vi "PKYK_Status.vi"(4 "QUpdate":bool=TRUE, 6 "PokaYoke?":bool, 8 "error in (no error)":errorcluster, 11 "Ref in":T5={"MS SQL Connection"=refnum, "UDL File"=path "", "Time"="", "DCODE"="", "WIP+1"=0, "MC No?"=0, "POKAYOKE?"=FALSE, "Expected Result"="", "Result [Status]"="", "Clock"=0.0, "RFID"="", "WIP Queue"=refnum, "TS Parameter"={"ProfitCenterCode"="", "LineCode"="", "WorkOrderNumber"="", "Model"="", "Model_with_Prefix"="", "VendorCode"="", "SetParameterDateCode"="", "PokaYoke"=0, "Target"=1, "Live_DateCode"="", "CustomerPartNumber"="", "Hand"="", "sBarcode"=FALSE, "FCA"=0, "Ent_Stamp"=timestamp(0 s since 1904-01-01), "STS_CD"=0.0}, "Data_Queue"=[], "RFID Serial No."=""} {"TS Parameter"."FCA" format="%01d"; "TS Parameter"."Target" min=1 max=100000; "TS Parameter"."PokaYoke" min=0 max=1}) -> (0 "error out":errorcluster, 2 "PKYK_Data Out":T1, 3 "Ref out":T5={"MS SQL Connection"=refnum, "UDL File"=path "", "Time"="", "DCODE"="", "WIP+1"=0, "MC No?"=0, "POKAYOKE?"=FALSE, "Expected Result"="", "Result [Status]"="", "Clock"=0.0, "RFID"="", "WIP Queue"=refnum, "TS Parameter"={"ProfitCenterCode"="", "LineCode"="", "WorkOrderNumber"="", "Model"="", "Model_with_Prefix"="", "VendorCode"="", "SetParameterDateCode"="", "PokaYoke"=0, "Target"=1, "Live_DateCode"="", "CustomerPartNumber"="", "Hand"="", "sBarcode"=FALSE, "FCA"=0, "Ent_Stamp"=timestamp(0 s since 1904-01-01), "STS_CD"=0.0}, "Data_Queue"=[], "RFID Serial No."=""} {"TS Parameter"."FCA" format="%01d"; "TS Parameter"."Target" min=1 max=100000; "TS Parameter"."PokaYoke" min=0 max=1}, 5 "Pky Status":T2)   [LabVIEW 2020]
uses:
  Controls/TD SQL.ctl
  <vilib>/addons/database/Connection.llb/Conn ObjectReference.ctl
  Controls/WIP_State.ctl
  Controls/TS_Parameter.ctl
  Controls/Poka_Status.ctl
  Controls/PKYK_qData.ctl
  Controls/PKYK_Barcode_Status.ctl
  Controls/PKYK_Status.ctl
  <vilib>/addons/database/NI_Database_API.lvlib
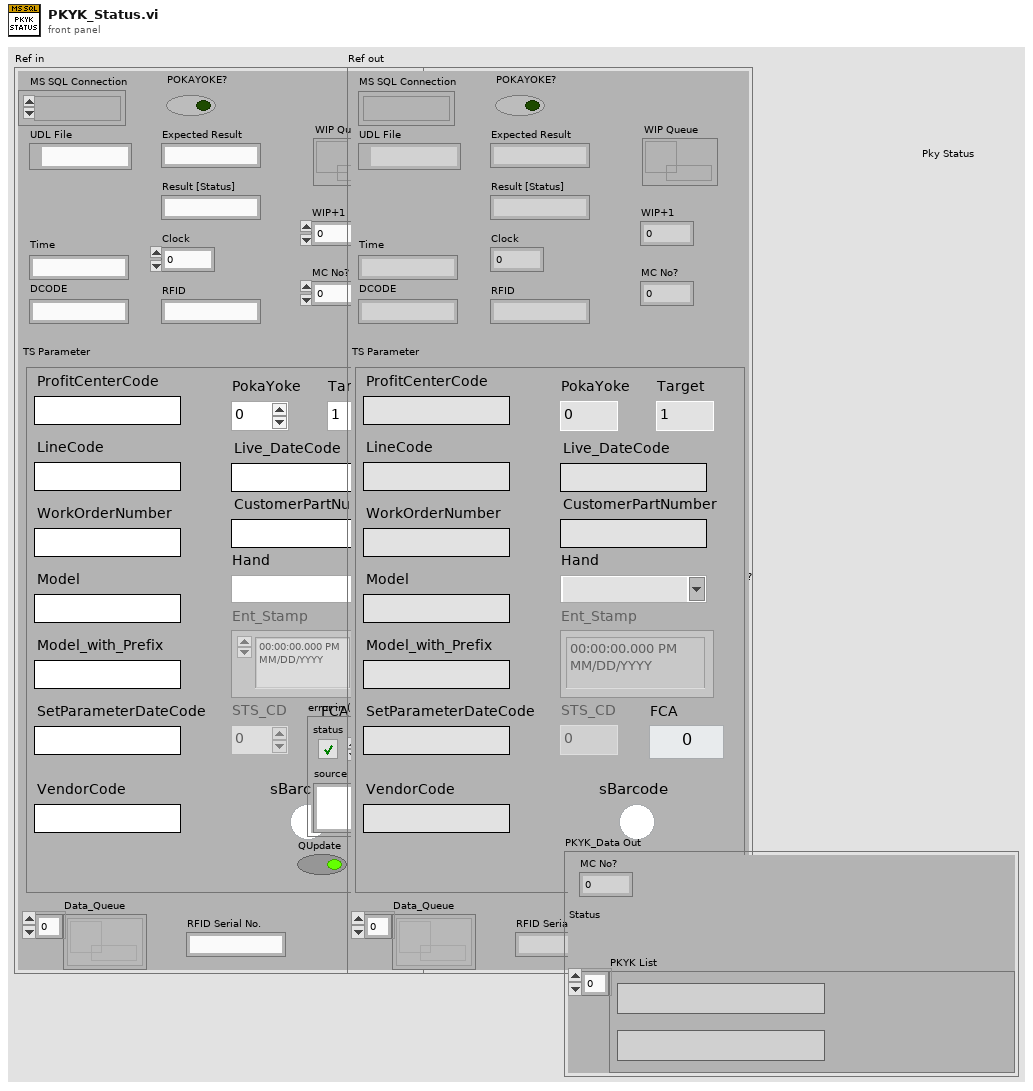
[diagram p1: front panel]
types:
  T1 = typedef "PKYK_qData.ctl" = cluster{"MC No?":i32, "Status":T2, "PKYK List":T3[]}
  T2 = typedef "Poka_Status.ctl" = u16
  T3 = typedef "PKYK_Barcode_Status.ctl" = cluster{"RFID Written Last":string, "Result":T4, "Exp. Result":T4}
  T4 = typedef "PKYK_Status.ctl" = u16
  T5 = typedef "TD SQL.ctl" = cluster{"MS SQL Connection":T6, "UDL File":path, "Time":string, "DCODE":string, "WIP+1":i64, "MC No?":i32, "POKAYOKE?":bool, "Expected Result":string, "Result [Status]":string, "Clock":dbl, "RFID":string, "WIP Queue":refnum<queue>, "TS Parameter":T7, "Data_Queue":refnum<queue>[], "RFID Serial No.":string}
  T6 = typedef "NI_Database_API.lvlib/Conn ObjectReference.ctl" = refnum<k1>
  T7 = typedef "TS_Parameter.ctl" = cluster{"ProfitCenterCode":string, "LineCode":string, "WorkOrderNumber":string, "Model":string, "Model_with_Prefix":string, "VendorCode":string, "SetParameterDateCode":string, "PokaYoke":i32, "Target":i32, "Live_DateCode":string, "CustomerPartNumber":string, "Hand":string, "sBarcode":bool, "FCA":i32, "Ent_Stamp":timestamp, "STS_CD":dbl}
  T8 = typedef "WIP_State.ctl" = enum16{"Open", "Read", "Write", "Read WIP", "Flush", "Close"}
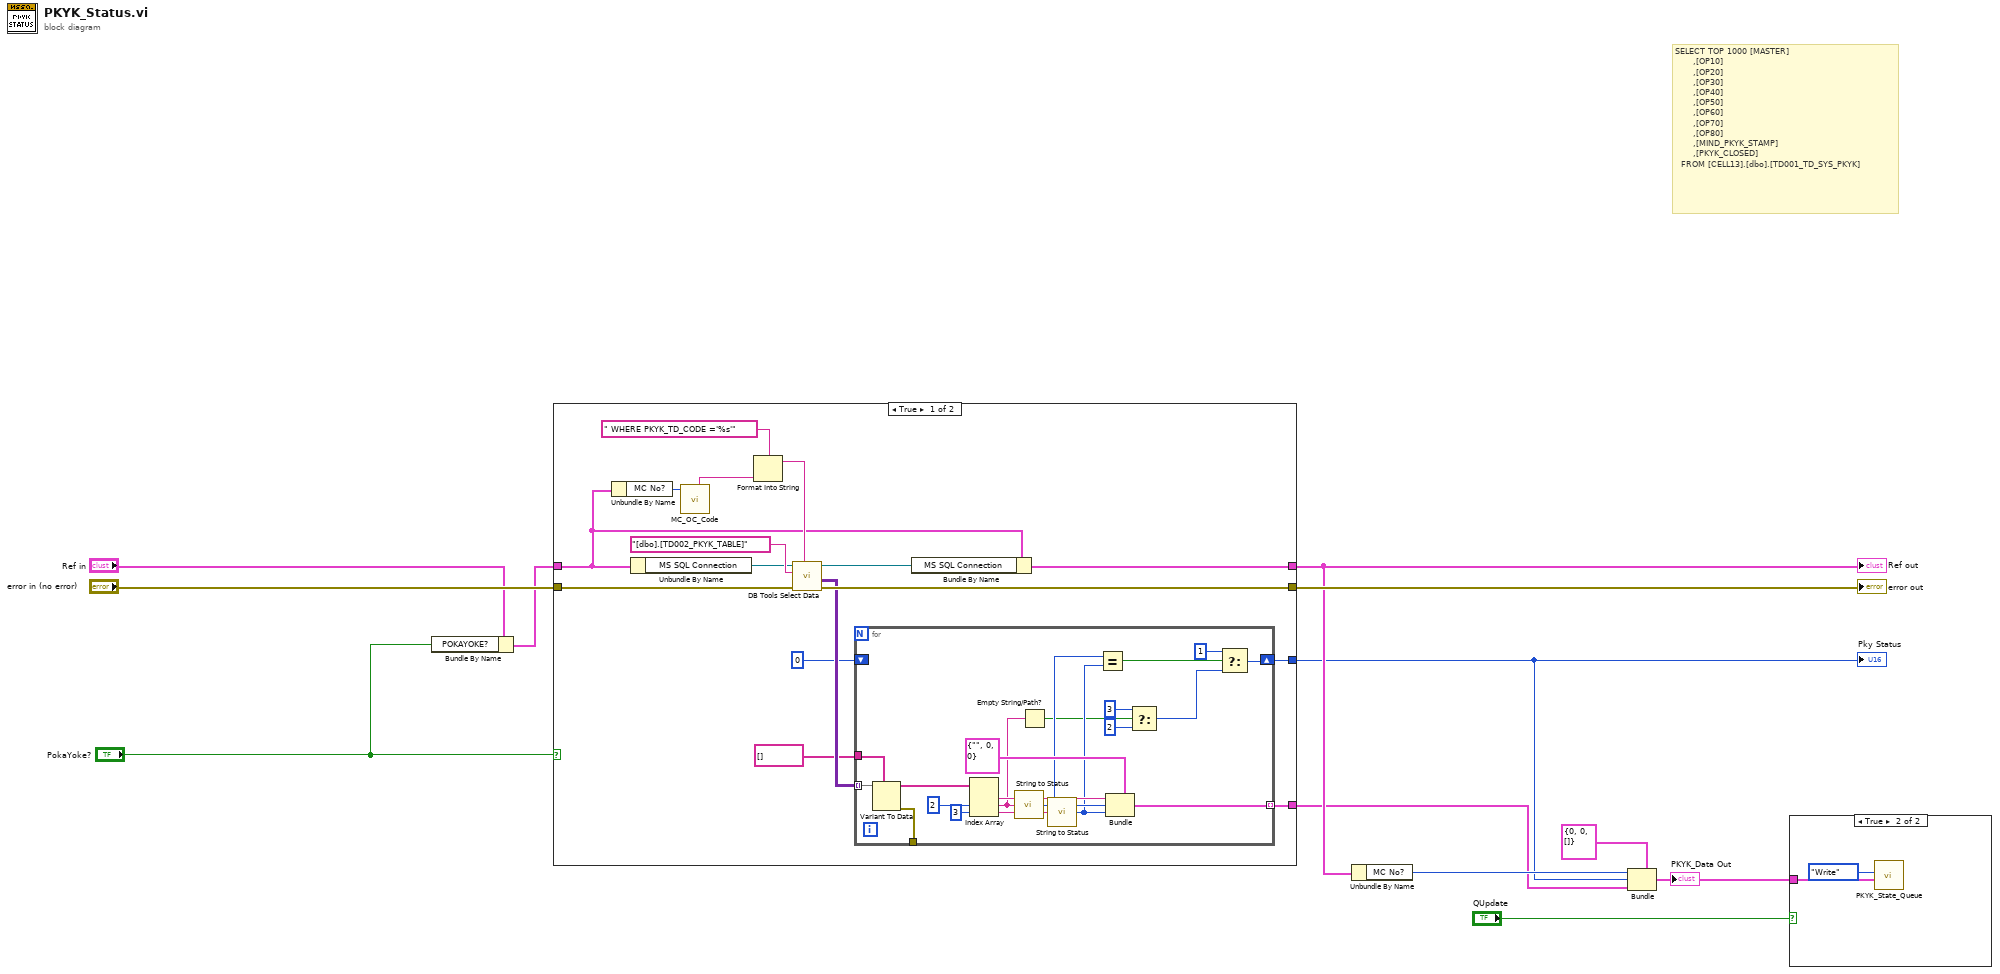
[diagram p0: block diagram]
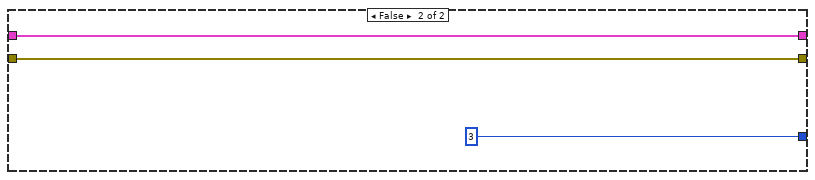
[diagram p3: hidden frame]
diagram:
  # "SELECT TOP 1000 [MASTER]\n      ,[OP10]\n      ,[OP20]\n      ,[OP30]\n      ,[OP40]\n      ,[OP50]\n      ,[OP60]\n      ,[OP70]\n      ,[OP80]\n      ,[MIND_PKYK_STAMP]\n      ,[PKYK_CLOSED]\n  FROM [CELL13].[dbo].[TD001_TD_SYS_PKYK]"
  n1 = Bundle By Name(cluster="Ref in", "POKAYOKE?"="PokaYoke?") -> (w10:T5)
  n2 = case shown="True" "PokaYoke?" {
    tunnel: [w28 w51] -> w8
    tunnel: [w26 w50] -> w11
    tunnel: "error in (no error)" -> [w23 w50]
    tunnel: w10 -> [w14 w51]
    tunnel: [w20 _] -> w6
    tunnel: [w16 T2 3 ("f")] -> w5
    frame True {
      n3 = Unbundle By Name(w14) -> ("MC No?"=w15:i32)
      n4 = Unbundle By Name(w14) -> ("MS SQL Connection"=w24:T6)
      n5 = call "MC_OC_Code.vi"("index"=w15) -> ("Machine No."=w13:string)  [unwired: 4 in, 6 out]
      n6 = Format Into String(format string=" WHERE PKYK_TD_CODE ='%s'", w13) -> (resulting string=w18:string)  [unwired: 2 in, 1 out]
      n7 = call <vilib>:"DB Tools Select Data.vi"("condition"=w18, "error in (no error)"=w23, "table"="[dbo].[TD002_PKYK_TABLE]", "connection reference"=w24) -> ("error out"=w26:errorcluster, "data"=w22:variant[][], "connection reference out"=w27:T6)  [unwired: 2 in]
      n8 = for {
        tunnel: w22 -> [w48] mode=indexing
        tunnel: string[] [] ("columns") -> [w47]
        tunnel: [w43] -> w20 mode=indexing
        tunnel: [w42] -> _
        shift-right: [w35] -> w16
        shift-left: T2 0 ("Pky Status") -> [_]
        n9 = Variant To Data(type=w47, Variant=w48) -> (data=w46:string[], error out=w42:errorcluster)  [unwired: 1 in]
        n10 = Index Array(array=w46, index #2=2 ("index"), index #3=3 ("index")) -> (element #1=w44:string, element #2=w31:string, element #3=w34:string)  [unwired: 1 in]
        n11 = call "String to Status.vi"("String"=w31) -> ("Result"=w39:T4)
        n12 = Empty String/Path?(string/path=w31) -> (empty?=w33:bool)
        n13 = call "String to Status.vi"("String"=w34) -> ("Result"=w38:T4)
        n14 = Equal?(x=w39, y=w38) -> (x = y?=w37:bool)
        n15 = Bundle(cluster=T3 {"RFID Written Last"="", "Result"=0, "Exp. Result"=0} ("PKYK Status"), "RFID Written Last"=w44, "Result"=w39, "Exp. Result"=w38) -> (w43:T3)
        n16 = Select(t=T2 3, s=w33, f=T2 2) -> (s? t:f=w29:T2)
        n17 = Select(t=T2 1, s=w37, f=w29) -> (s? t:f=w35:T2)
      }
      n18 = Bundle By Name(cluster=w14, "MS SQL Connection"=w27) -> (w28:T5)
    }
    frame False {
    }
  }
  "error out" <- w11
  "Ref out" <- w8
  "Pky Status" <- w5
  n19 = Unbundle By Name(w8) -> ("MC No?"=w7:i32)
  n20 = Bundle(cluster=T1 {"MC No?"=0, "Status"=0, "PKYK List"=[]} ("output cluster"), "MC No?"=w7, "Status"=w5, "PKYK List"=w6) -> (w3:T1)
  "PKYK_Data Out" <- w3
  n21 = case shown="True" "QUpdate" {
    tunnel: w3 -> [_ w53]
    frame False {
    }
    frame True {
      n22 = call "PKYK_State_Queue.vi"("PKYK_Data In"=w53, "State In"=WIP_State."Write") -> ()  [unwired: 7 in, 3 out]
    }
  }
